vi "Cleanup.vi"(8 "error in (no error)":errorcluster, 11 "WAMP Client in":refnum<class "WAMP Client.lvclass">) -> (0 "error out":errorcluster, 3 "WAMP Client out":refnum<class "WAMP Client.lvclass">)   [LabVIEW 2020, in "wamplv.lvlib" / "WAMP Client.lvclass"]
uses:
  <vilib>/samangh/wamplv/WAMP Client/WAMP Client.lvclass
  <vilib>/samangh/wamplv/WAMP Client/WAMP Client.lvclass/WAMP Client.ctl
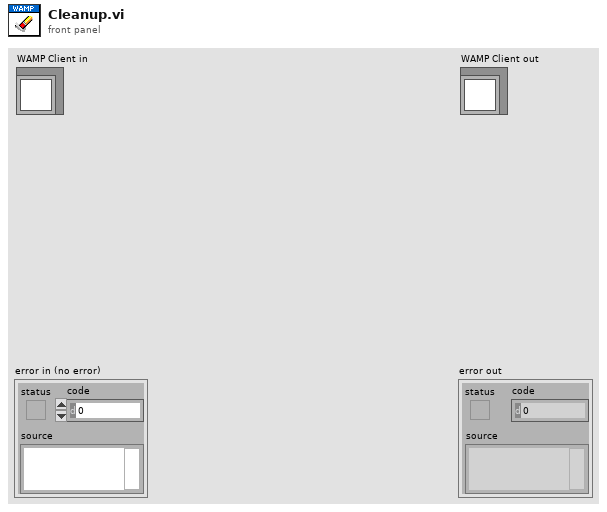
[diagram p1: front panel]
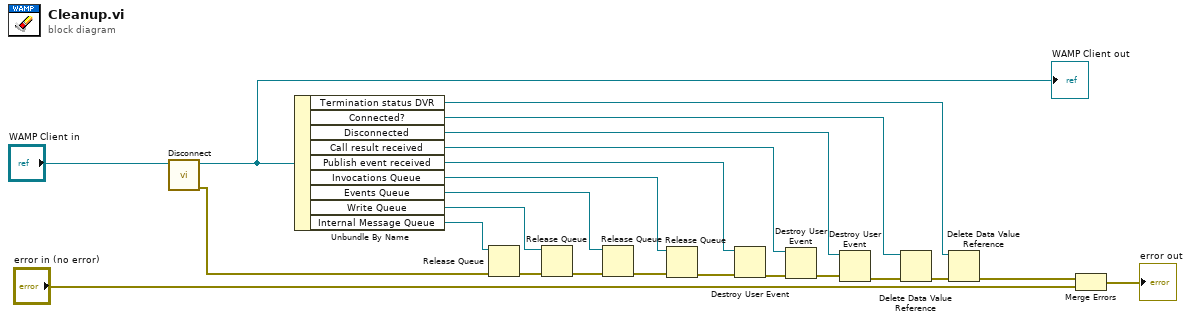
[diagram p0: block diagram]
diagram:
  n1 = call-dynamic "Disconnect.vi"("WAMP Client in"="WAMP Client in") -> ("error out"=w4:errorcluster, "WAMP Client out"=w5:refnum<class "WAMP Client.lvclass">)  [unwired: 9 in]
  "WAMP Client out" <- w5
  n2 = Unbundle By Name(w5) -> ("Termination status DVR"=w2:refnum<data-value>, "Connected?"=w17:refnum<data-value>, "Disconnected"=w20:refnum<user-event>, "Call result received"=w21:refnum<user-event>, "Publish event received"=w22:refnum<user-event>, "Invocations Queue"=w16:refnum<queue>, "Events Queue"=w15:refnum<queue>, "Write Queue"=w8:refnum<queue>, "Internal Message Queue"=w7:refnum<queue>)
  n3 = Release Queue(queue=w7, error in (no error)=w4) -> (error out=w9:errorcluster)  [unwired: 1 in, 2 out]
  n4 = Release Queue(queue=w8, error in (no error)=w9) -> (error out=w10:errorcluster)  [unwired: 1 in, 2 out]
  n5 = Release Queue(queue=w15, error in (no error)=w10) -> (error out=w13:errorcluster)  [unwired: 1 in, 2 out]
  n6 = Release Queue(queue=w16, error in (no error)=w13) -> (error out=w14:errorcluster)  [unwired: 1 in, 2 out]
  n7 = Destroy User Event(user event=w22, error in=w14) -> (error out=w23:errorcluster)
  n8 = Destroy User Event(user event=w21, error in=w23) -> (error out=w19:errorcluster)
  n9 = Destroy User Event(user event=w20, error in=w19) -> (error out=w18:errorcluster)
  n10 = Delete Data Value Reference(data value reference=w17, error in=w18) -> (error out=w3:errorcluster)  [unwired: 1 out]
  n11 = Delete Data Value Reference(data value reference=w2, error in=w3) -> (error out=w1:errorcluster)  [unwired: 1 out]
  n12 = Merge Errors(w1, "error in (no error)") -> (→"error out":errorcluster)
